vi "Write Pulse File.vi"(8 "error in (no error)":errorcluster, 9 "Open plot after pulse":bool, 10 "Pulse File":path, 11 "Monitor-Pulse in":refnum<class "LabActor.lvclass">) -> (0 "error out":errorcluster, 3 "Monitor-Pulse out":refnum<class "LabActor.lvclass">)   [LabVIEW 2021, in "LabActor.lvclass"]
uses:
  LabActor.lvclass
  C:/GitHub/LabActor/Template Module/Template Module.lvclass
  Plots/Plot types.ctl
  NHMFL_Core/Libraries/Instruments/Results/File Path Result/File Path Result.lvclass
  C:/GitHub/NHMFL_Core/Libraries/Instruments/Results/Acquired Result/Acquired Result.lvclass
  Template Module/Template Module.lvclass/Template Module.ctl
  NHMFL_Core/Libraries/Instruments/Results/Acquired Result/Acquired Result.lvclass/Acquired Result.ctl
  Template Module/Read Name.vi
  NHMFL_Core/Libraries/Instruments/Results/Acquired Result/Write Sender.vi
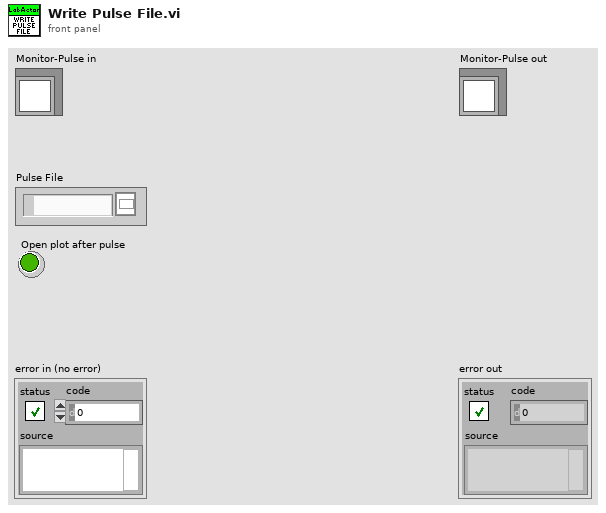
[diagram p1: front panel]
types:
  T1 = typedef "Plot types.ctl" = enum16{"Waveform Plot", "XY Plot", "Full XY"}
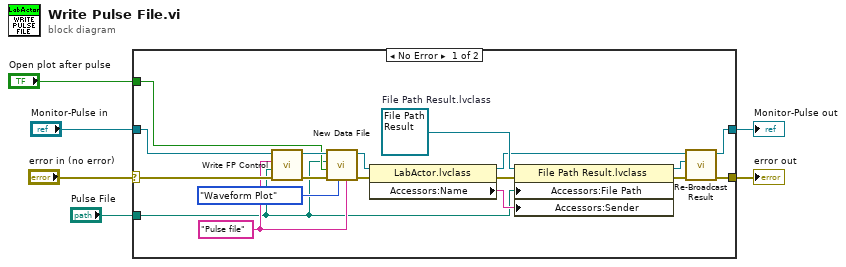
[diagram p0: block diagram]
diagram:
  n1 = case shown="No Error" "error in (no error)" {
    selector: "error in (no error)" -> [w23 w26]
    tunnel: [w10 w26] -> w5
    tunnel: [w8 w25] -> w3
    tunnel: "Monitor-Pulse in" -> [w24 w25]
    tunnel: "Open plot after pulse" -> [w18 _]
    tunnel: "Pulse File" -> [w7 _]
    frame No Error {
      w17 = refnum<class "File Path Result.lvclass"> refnum  # File Path Result.lvclass
      w19 = "Pulse file" ("Control Name")
      n2 = call-dynamic "Write FP Control.vi"("error in (no error)"=w23, "Control Value"=w7, "Control Name"=w19, "Measure Object in"=w24) -> ("error out"=w21:errorcluster, "Measure Object out"=w22:refnum<class "LabActor.lvclass">)  [unwired: 6 in]
      n3 = call-dynamic "New Data File.vi"("Plot group"=w19, "Plot type"=Plot_types."Waveform Plot", "error in (no error)"=w21, "New plot if not open"=w18, "File"=w7, "Application Controller in"=w22) -> ("error out"=w11:errorcluster, "Application Controller out"=w9:refnum<class "LabActor.lvclass">)  [unwired: 4 in]
      n4 = property class="LabActor.lvclass"(reference=w9, error in=w11) -> (reference out=w13:refnum<class "LabActor.lvclass">, error out=w15:errorcluster, "Accessors:Name"=w16:string)
      n5 = property class="File Path Result.lvclass"(reference=w17, error in=w15, "Accessors:File Path"=w7, "Accessors:Sender"=w16) -> (reference out=w14:refnum<class "File Path Result.lvclass">, error out=w12:errorcluster)
      n6 = call-dynamic "Re-Broadcast Result.vi"("error in (no error)"=w12, "Acquired Result.lvclass"=w14, "Measure Object in"=w13) -> ("error out"=w10:errorcluster, "Measure Object out"=w8:refnum<class "LabActor.lvclass">)  [unwired: 7 in]
    }
    frame Error {
    }
  }
  "error out" <- w5
  "Monitor-Pulse out" <- w3
